vi "Set Variable Value.vi"(8 "error in (no error)":errorcluster, 9 "VAR Value":string, 10 "VAR NAME":string, 11 "Domino Laser module Class in":refnum<class "Domino Laser module Class.lvclass">) -> (0 "error out":errorcluster, 2 "Var changed successfully?":bool, 3 "Domino Laser module Class out":refnum<class "Domino Laser module Class.lvclass">)   [LabVIEW 2015, in "Domino LM.lvlib" / "Domino Laser module Class.lvclass"]
uses:
  CTRLS/Domino Laser module Class.lvclass
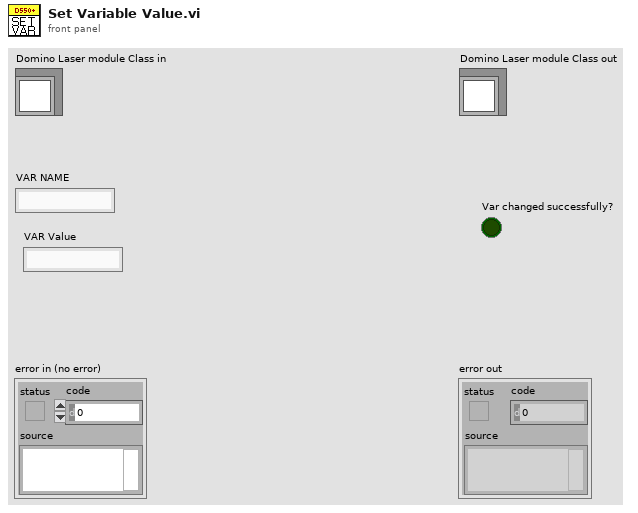
[diagram p1: front panel]
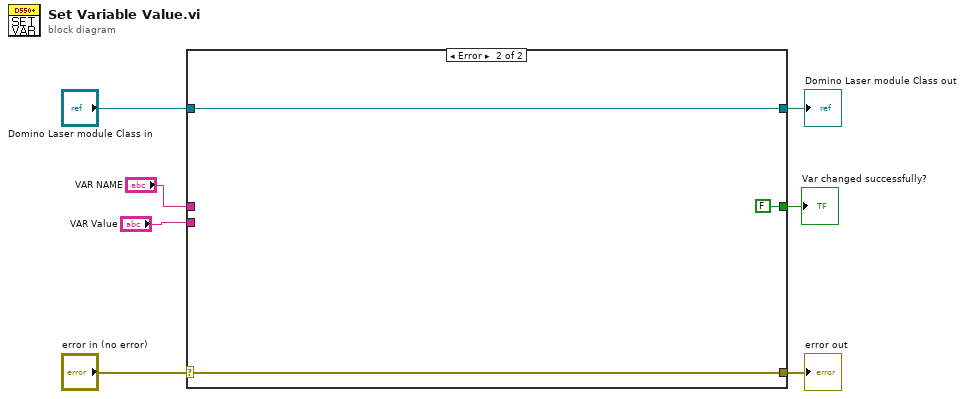
[diagram p0: block diagram]
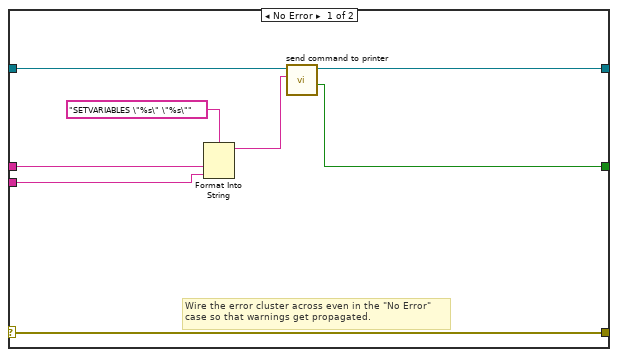
[diagram p2: hidden frame]
diagram:
  n1 = case shown="Error" "error in (no error)" {
    selector: "error in (no error)" -> [w15 w18]
    tunnel: [w15 w18] -> w6
    tunnel: [w13 w17] -> w4
    tunnel: "Domino Laser module Class in" -> [w14 w17]
    tunnel: "VAR NAME" -> [w11 _]
    tunnel: "VAR Value" -> [w10 _]
    tunnel: [w8 FALSE ("Command Excuted succeddfully?")] -> w1
    frame No Error {
      # "Wire the error cluster across even in the \"No Error\"\ncase so that warnings get propagated."
      n2 = Format Into String(format string="SETVARIABLES \"%s\" \"%s\"", w11, w10) -> (resulting string=w9:string)  [unwired: 2 in, 1 out]
      n3 = call "send command to printer.vi"("command to be sent"=w9, "Domino Laser module Class in"=w14) -> ("Command Excuted succeddfully?"=w8:bool, "Domino Laser module Class out"=w13:refnum<class "Domino Laser module Class.lvclass">)  [unwired: 6 in, 2 out]
    }
    frame Error {
    }
  }
  "error out" <- w6
  "Domino Laser module Class out" <- w4
  "Var changed successfully?" <- w1
